vi "L06.vi"() -> ()   [LabVIEW 2012]
panel:
  out "x-y":i32
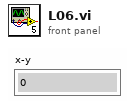
[diagram p1: front panel]
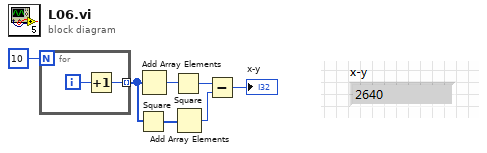
[diagram p0: block diagram]
diagram:
  n1 = for {
    N: 10 -> [_]
    tunnel: [w8] -> w4 mode=indexing
    i -> [w9]
    n2 = Increment(x=w9) -> (x+1=w8:i32)
  }
  n3 = Square(x=w4) -> (x^2=w6:i32[])
  n4 = Add Array Elements(numeric array=w4) -> (sum=w5:i32)
  n5 = Square(x=w5) -> (x^2=w3:i32)
  n6 = Add Array Elements(numeric array=w6) -> (sum=w2:i32)
  n7 = Subtract(x=w3, y=w2) -> (x-y=→"x-y":i32)
